vi "StartAsynchroneVi.vi"(6 "Open Front Panel ?":bool, 7 "EVE reference in":refnum<data-value>, 8 "error in":errorcluster, 9 "State":T1(ring), 10 "viInitString":string, 11 "viPathToStart":path) -> (0 "error out":errorcluster, 3 "vi reference":refnum<vi>)   [LabVIEW 2013]
uses:
  001 - MAIN/Class/EVE/EVE.lvclass
  001 - MAIN/Class/EVE/Process_Proto.ctl
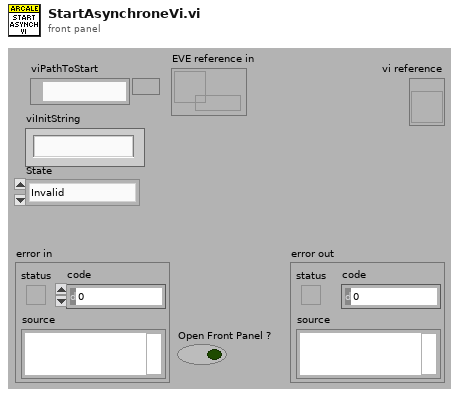
[diagram p1: front panel]
types:
  T1 = enum32{"Invalid", "Standard", "Closed", "Hidden", "Minimized", "Maximized"}
  T2 = typedef "EVE.lvclass/Process_Proto.ctl" = refnum<vi>
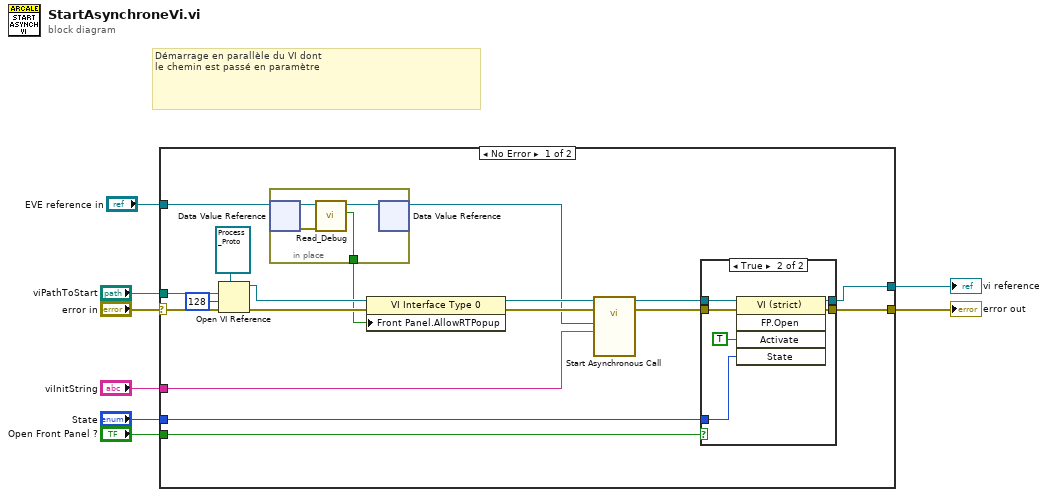
[diagram p0: block diagram]
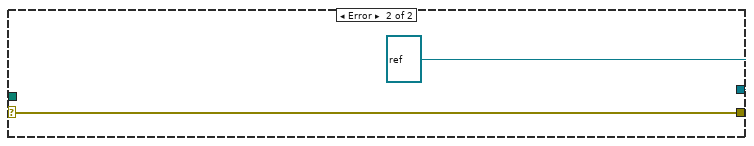
[diagram p3: hidden frame]
diagram:
  # "Démarrage en parallèle du VI dont\nle chemin est passé en paramètre"
  n1 = case shown="No Error" "error in" {
    selector: "error in" -> [w22 w40]
    tunnel: [w26 w40] -> w8
    tunnel: [w25 refnum<vi> refnum ("vi reference")] -> w7
    tunnel: "Open Front Panel ?" -> [w21 _]
    tunnel: "viPathToStart" -> [w19 _]
    tunnel: "viInitString" -> [w9 _]
    tunnel: "State" -> [w20 _]
    tunnel: "EVE reference in" -> [w18 _]
    frame No Error {
      n2 = Open VI Reference(type specifier VI Refnum (for type only)=T2 refnum ("Process Prototype"), vi path=w19, options=128, error in (no error)=w22) -> (vi reference=w23:T2, error out=w24:errorcluster)  [unwired: 2 out]
      n3 = in-place {
        in-place-border: [w28] -> w13
        n4 = in-place-dvr #1(w18) -> (w30:refnum<class "EVE.lvclass">, w27:errorcluster)
        n5 = call-dynamic "Read_Debug.vi"("error in (no error)"=w27, "EVE in"=w30) -> ("Debug ?"=w28:bool, "EVE out"=w29:refnum<class "EVE.lvclass">)  [unwired: 7 in, 1 out]
        n6 = in-place-dvr #1(w29) -> (w10:refnum<data-value>)  [unwired: 1 out]
      }
      n7 = property class="VI Interface Type 0"(reference=w23, error in=w24, "Front Panel.AllowRTPopup"=w13) -> (reference out=w12:T2, error out=w16:errorcluster)
      n8 = call-by-ref "Start Asynchronous Call"(reference=w12, error in=w16, "InitString"=w9, "EVE reference in"=w10) -> (reference out=w15:T2, error out=w14:errorcluster)  [unwired: 10 in]
      n9 = case shown="True" w21 {
        tunnel: w15 -> [w32 w38]
        tunnel: w14 -> [w31 w37]
        tunnel: [w31 w36] -> w26
        tunnel: [w32 w35] -> w25
        tunnel: w20 -> [_ w33]
        frame False {
        }
        frame True {
          n10 = invoke class="VI (strict)" method="FP.Open"(reference=w38, error in=w37, "Activate"=TRUE ("Activate?"), "State"=w33) -> (reference out=w35:T2, error out=w36:errorcluster)  [unwired: 1 in, 3 out]
        }
      }
    }
    frame Error {
    }
  }
  "error out" <- w8
  "vi reference" <- w7
